vi "Set Detection.vi"(8 "error in (no error)":errorcluster, 10 "Detection":T1=enum."Cy3 (LP550)", 11 "TE2000 in":refnum<class "TE2000.lvclass">) -> (0 "error out":errorcluster, 3 "TE2000 out":refnum<class "TE2000.lvclass">)   [LabVIEW 2014, in "TE2000.lvlib" / "TE2000.lvclass"]
uses:
  TE2000.lvclass
  Resources/Type Defs/Detection.ctl
  TE2000.lvclass/TE2000.ctl
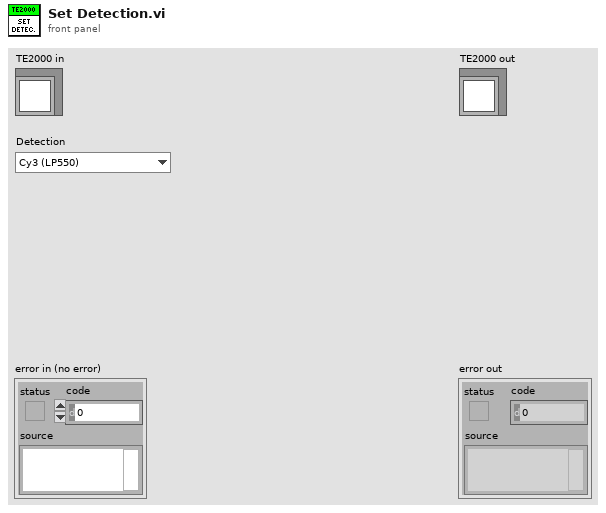
[diagram p1: front panel]
types:
  T1 = typedef "Detection.ctl" = enum16{"Cy2 (LP500)", "Cy3 (LP550)", "Cy5 (BP700/75)", "Cy3/Cy5 (BP590/40,700/60)", "No Filter", "Laser to Eyes"}
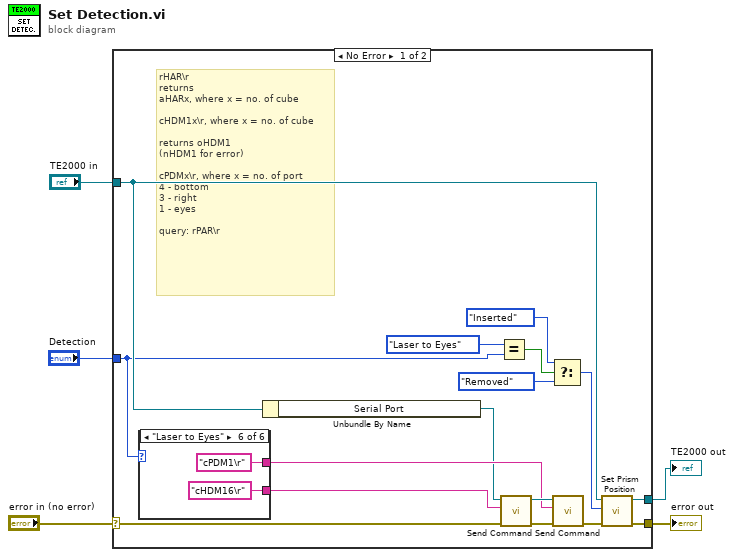
[diagram p0: block diagram]
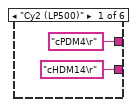
[diagram p2: hidden frame]
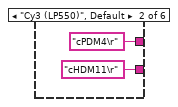
[diagram p3: hidden frame]
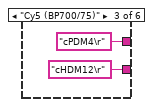
[diagram p4: hidden frame]
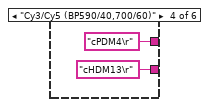
[diagram p5: hidden frame]
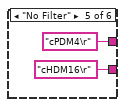
[diagram p6: hidden frame]
diagram:
  n1 = case shown="No Error" "error in (no error)" {
    selector: "error in (no error)" -> [w21 w35]
    tunnel: [w14 w35] -> w4
    tunnel: [w12 w34] -> w2
    tunnel: "TE2000 in" -> [w13 w34]
    tunnel: "Detection" -> [w11 _]
    frame No Error {
      # "rHAR\\r\nreturns\naHARx, where x = no. of cube\n\ncHDM1x\\r, where x = no. of cube\n\nreturns oHDM1\n(nHDM1 for error)\n\ncPDMx\\r, where x = no. of port\n4 - bottom\n3 - right\n1 - eyes\n\nquery: rPAR\\r"
      n2 = case shown="\"Laser to Eyes\"" w11 {
        tunnel: ["cHDM14\r" "cHDM11\r" "cHDM12\r" "cHDM13\r" "cHDM16\r" "cHDM16\r"] -> w18
        tunnel: ["cPDM4\r" "cPDM4\r" "cPDM4\r" "cPDM4\r" "cPDM4\r" "cPDM1\r"] -> w17
        frame "Cy2 (LP500)" {
        }
        frame "Cy3 (LP550)", Default {
        }
        frame "Cy5 (BP700/75)" {
        }
        frame "Cy3/Cy5 (BP590/40,700/60)" {
        }
        frame "No Filter" {
        }
        frame "Laser to Eyes" {
        }
      }
      n3 = Unbundle By Name(w13) -> ("Serial Port"=w16:refnum<visa-resource-name>)
      n4 = Equal?(x=Detection."Laser to Eyes", y=w11) -> (x = y?=w9:bool)
      n5 = call "Send Command.vi"("error in (no error)"=w21, "Command"=w18, "Serial Port In"=w16) -> ("error out"=w20:errorcluster, "Serial Port Out"=w19:refnum<visa-resource-name>)  [unwired: 6 in, 1 out]
      n6 = Select(t=enum16{"Removed", "Inserted"}."Inserted" ("Prism Position"), s=w9, f=enum16{"Removed", "Inserted"}."Removed" ("Prism Position")) -> (s? t:f=w6:enum16{"Removed", "Inserted"})
      n7 = call "Send Command.vi"("error in (no error)"=w20, "Command"=w17, "Serial Port In"=w19) -> ("error out"=w15:errorcluster)  [unwired: 6 in, 2 out]
      n8 = call-dynamic "Set Prism Position.vi"("error in (no error)"=w15, "Prism Position"=w6, "TE2000 in"=w13) -> ("error out"=w14:errorcluster, "TE2000 out"=w12:refnum<class "TE2000.lvclass">)  [unwired: 7 in]
    }
    frame Error {
    }
  }
  "error out" <- w4
  "TE2000 out" <- w2
